vi "ICM Open Bus.vi"(8 "error in (no error)":errorcluster, 11 "ICM File In":path) -> (0 "error out":errorcluster, 3 "Bus out":refnum<class "Bus.lvclass">)   [LabVIEW 2024]
doc: "ICM Open Bus.vi\n\nThis VI finds the Bus of the current configuration file, opens the object, and reads its configuration data.\n\nInstrument Communication Module Version 1.0\nSeptember, 2017 Original Code Consulting David Thomson\n www.originalcode.com"
uses:
  Bus/Bus.lvclass
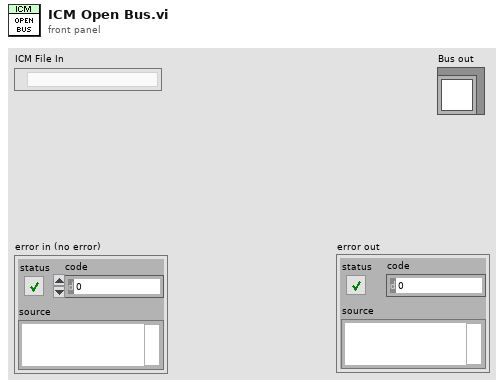
[diagram p1: front panel]
types:
  T1 = enum32{"invalid app kind", "Development System", "Run Time System", "Student Edition", "Embedded LabVIEW", "Evaluation", "Custom"}
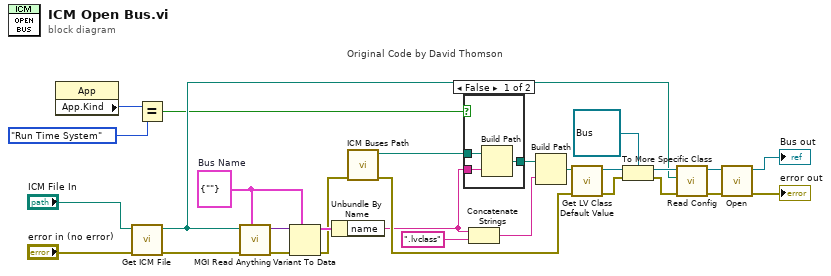
[diagram p0: block diagram]
diagram:
  w26 = cluster{"name":string} {"name"=""}  # Bus Name
  n1 = property class="App"() -> ("App.Kind"=w3:T1)  [unwired: 2 in, 2 out]
  n2 = call "Get ICM File.vi"("error in (no error)"="error in (no error)", "ICM File In"="ICM File In") -> ("error out"=w19:errorcluster, "ICM File"=w9:path)  [unwired: 8 in]
  n3 = Equal?(x=w3, y=T1."Run Time System" ("Application:Kind")) -> (x = y?=w1:bool)
  n4 = call <userlib>:"MGI Read Anything.vi"("Type of Anything"=w26, "Error In"=w19, "Path (dialog)"=w9) -> ("Error Out"=w28:errorcluster, "Anything"=w27:variant)  [unwired: 5 in, 2 out]
  n5 = Variant To Data(error in=w28, type=w26, Variant=w27) -> (data=w22:cluster{"name":string}, error out=w7:errorcluster)
  n6 = Unbundle By Name(w22) -> ("name"=w6:string)
  n7 = call "ICM Buses Path.vi"("error in (no error)"=w7) -> ("error out"=w8:errorcluster, "ICM Buses Path"=w4:path)  [unwired: 9 in]
  n8 = case "Original Code by David Thomson" shown="False" w1 {
    tunnel: w4 -> [w31 w32]
    tunnel: [w30 w32] -> w5
    tunnel: w6 -> [w29 _]
    frame False {
      n9 = Build Path(base path=w31, name or relative path=w29) -> (appended path=w30:path)
    }
    frame True {
    }
  }
  n10 = Concatenate Strings(w6, ".lvclass" ("string")) -> (w23:string)
  n11 = Build Path(base path=w5, name or relative path=w23) -> (appended path=w25:path)
  n12 = call <vilib>:"Get LV Class Default Value.vi"("error in (no error)"=w8, "class path"=w25) -> ("error out"=w21:errorcluster, "object"=w20:refnum<class>)  [unwired: 8 in]
  n13 = To More Specific Class(target class=refnum<class "Bus.lvclass"> refnum ("Bus.lvclass"), reference=w20, error in=w21) -> (specific class reference=w16:refnum<class "Bus.lvclass">, error out=w15:errorcluster)
  n14 = call-dynamic "Read Config.vi"("error in (no error)"=w15, "ICM File In"=w9, "Bus in"=w16) -> ("error out"=w13:errorcluster, "Bus out"=w14:refnum<class "Bus.lvclass">)  [unwired: 7 in]
  n15 = call-dynamic "Open.vi"("error in (no error)"=w13, "Bus in"=w14) -> ("error out"=→"error out":errorcluster, "Bus out"=→"Bus out":refnum<class "Bus.lvclass">)  [unwired: 8 in]
